vi "Duplicate.vi"(8 "error in":errorcluster, 10 "parameters":variant, 11 "CEF_Serialize node in":refnum<class "CEF_serializable node.lvclass">) -> (0 "error out":errorcluster, 3 "CEF_Serialize node out":refnum<class "CEF_serializable node.lvclass">)   [LabVIEW 2025, in "CEF.lvlib" / "CEF_serializable node.lvclass"]
doc: "Implements the specific behavior of a node when it is being duplicated\nCan be used to change the name of the new node for example adding Copy to it. \nCopyright 2017 National Instruments Corporation\n\nLicensed under the Apache License, Version 2.0 (the \"License\"); you may not use this file except in compliance with the License. You may obtain a copy of the License at http://www.apache.org/licenses/LICENSE-2.0\nUnless required by applicable law or agreed to in writing, software distributed under the License is distributed on an \"AS IS\" BASIS, WITHOUT WARRANTIES OR CONDITIONS OF ANY KIND, either express or implied. See the License for the specific language governing permissions and limitations under the License."
uses:
  CEF_serializable node.lvclass
  serializable configuration/CEF_serializable configuration.lvclass
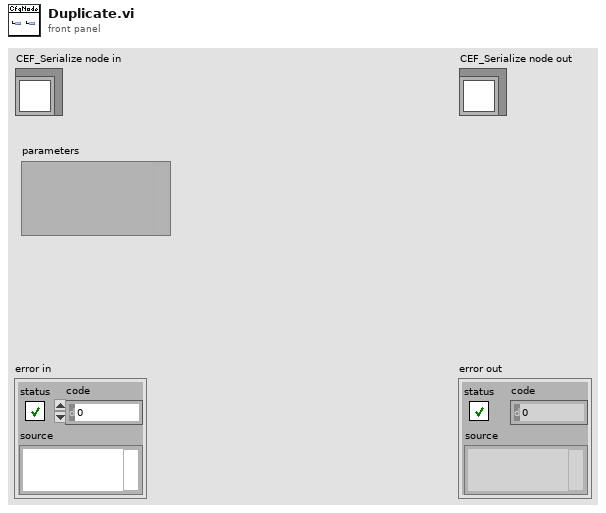
[diagram p1: front panel]
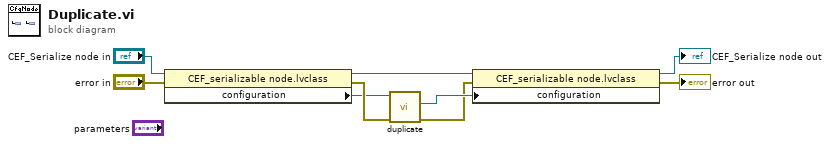
[diagram p0: block diagram]
diagram:
  n1 = property class="CEF_serializable node.lvclass"(reference="CEF_Serialize node in", error in="error in") -> (reference out=w3:refnum<class "CEF_serializable node.lvclass">, error out=w5:errorcluster, "configuration"=w4:refnum<class "CEF_serializable configuration.lvclass">)
  n2 = call-dynamic "duplicate.vi"("error in"=w5, "CEF_Configuration in"=w4) -> ("error out"=w1:errorcluster, "duplicate configuration out"=w2:refnum<class "CEF_serializable configuration.lvclass">)  [unwired: 7 in, 1 out]
  n3 = property class="CEF_serializable node.lvclass"(reference=w3, error in=w1, "configuration"=w2) -> (reference out=→"CEF_Serialize node out":refnum<class "CEF_serializable node.lvclass">, error out=→"error out":errorcluster)
